vi "RegisterImageRoutedMessage_Name.vi"() -> (1 "message name":string="IrDataEventCreator.RegisterImage")   [LabVIEW 2017, in "IrDataEventCreator.lvlib"]
uses:
  <vilib>/addons/InsightCM/Devices/Shared/Ir/IrDataEventCreator/IrDataEventCreator.lvlib
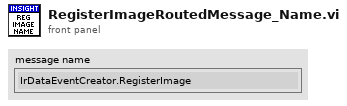
[diagram p1: front panel]
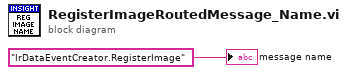
[diagram p0: block diagram]
diagram:
  "message name" <- "IrDataEventCreator.RegisterImage"
